vi "FT_Read_Byte_Data.vi"(0 "Handle":u32, 1 "Bytes To Read":u32) -> (2 "FT_Status":u32(ring) items=["FT_OK", "FT_INVALID_HANDLE", "FT_DEVICE_NOT_FOUND", "FT_DEVICE_NOT_OPENED", "FT_IO_ERROR", "FT_INSUFFICIENT_RESOURCES", "FT_INVALID_PARAMETER", "FT_INVALID_BAUD_RATE", "FT_DEVICE_NOT_OPENED_FOR_ERASE", "FT_DEVICE_NOT_OPENED_FOR_WRITE", "FT_FAILED_TO_WRITE_DEVICE", "FT_EEPROM_READ_FAILED", "FT_EEPROM_WRITE_FAILED", "FT_EEPROM_ERASE_FAILED", "FT_EEPROM_NOT_PRESENT", "FT_EEPROM_NOT_PROGRAMMED", "FT_INVALID_ARGS", "FT_NOT_SUPPORTED", "FT_OTHER_ERROR"], 3 "Read Data":u8[](array[numeric]), 4 "Bytes Read":u32)   [LabVIEW 2020]
uses:
  GEA3 DLL Source/ftd2xx.dll
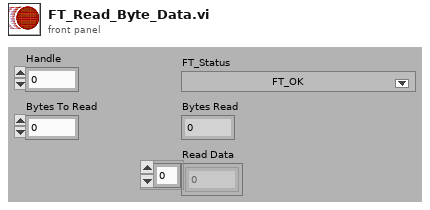
[diagram p1: front panel]
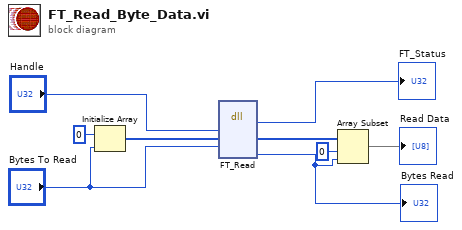
[diagram p0: block diagram]
diagram:
  n1 = Initialize Array(u8 0 ("element"), "Bytes To Read") -> (w7:u8[])
  n2 = dll-call lib="C:/TechnologyLab/NI-2010/Drivers/GEA3 Toolkit/GEA3 DLL Source/FTD2XX.dll" fn="FT_Read"("Handle"="Handle", "Buffer"=w7, "BytesToRead"="Bytes To Read") -> ("FT_Status"=→"FT_Status":u32, "Buffer"=w4:u8[], "BytesReturned"=w2:u32)  [unwired: 6 in, 2 out]
  "Bytes Read" <- w2
  n3 = Array Subset(array=w4, index=0, length=w2) -> (→"Read Data":u8[])
